vi "SkipStepHandle.vi"(9 "ItemNamesIn":string[][](array[string]), 11 "ShowSkipStep?":bool) -> (1 "ItemNamesOut":string[][](array[string]))   [LabVIEW 2013]
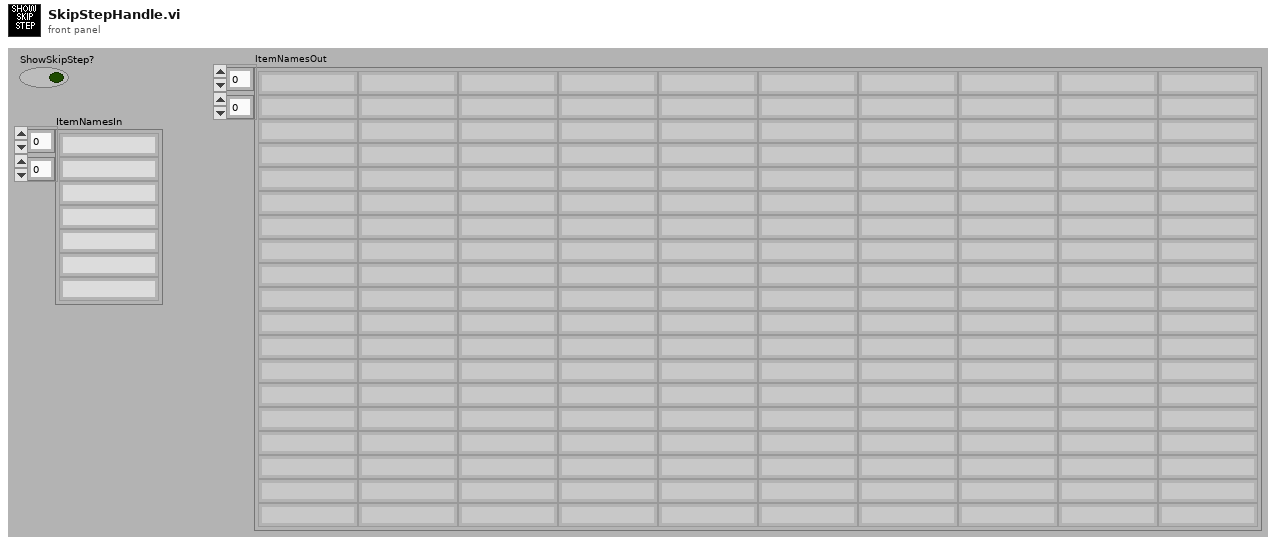
[diagram p1: front panel]
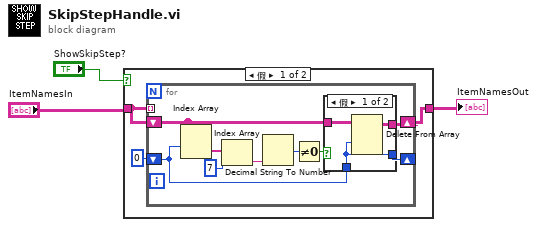
[diagram p0: block diagram]
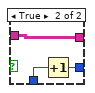
[diagram p2: hidden frame]
diagram:
  n1 = case shown="假" "ShowSkipStep?" {
    tunnel: "ItemNamesIn" -> [w6 w22]
    tunnel: [w5 w22] -> w3
    frame False {
      n2 = for {
        tunnel: w6 -> [_] mode=indexing
        shift-right: [w15] -> w5
        shift-left: w6 -> [w10]
        shift-right: [w7] -> _
        shift-left: 0 ("index") -> [w8]
        n3 = Index Array(array=w10, index (row)=w8) -> (element=w9:string[])  [unwired: 1 in]
        n4 = Index Array(array=w9, index=7) -> (element=w12:string)
        n5 = Decimal String To Number(string=w12) -> (number=w11:i32)  [unwired: 3 out]
        n6 = Not Equal To 0?(x=w11) -> (x != 0?=w14:bool)
        n7 = case shown="假" w14 {
          tunnel: w10 -> [w18 w21]
          tunnel: [w17 w21] -> w15
          tunnel: w8 -> [w16 w20]
          tunnel: [w16 w19] -> w7
          frame False {
            n8 = Delete From Array(array=w18, index (row)=w16) -> (array with subset deleted=w17:string[][])  [unwired: 2 in, 1 out]
          }
          frame True {
            n9 = Increment(x=w20) -> (x+1=w19:i32)
          }
        }
      }
    }
    frame True {
    }
  }
  "ItemNamesOut" <- w3
